vi "FPGA_measure_loop_time.vi"() -> (3 "Numeric":u32)   [LabVIEW 2020]
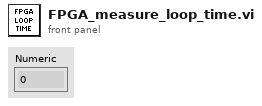
[diagram p1: front panel]
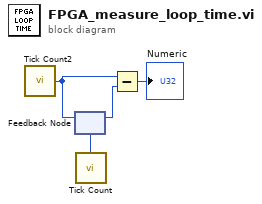
[diagram p0: block diagram]
diagram:
  n1 = call "Tick Count2"() -> ("Tick Count(Ticks)"=w2:u32)
  n2 = feedback-in #1(w2) -> ()
  n3 = call "Tick Count"() -> ("Tick Count(Ticks)"=w1:u32)
  n4 = feedback #1(w1) -> (w3:u32)
  n5 = Subtract(x=w2, y=w3) -> (x-y=→"Numeric":u32)
